vi "XY Graph Select Plots... Event.vi"(8 "Error In":errorcluster, 10 "Select (T)/Deselect":bool=TRUE, 11 "XYGraph Ref":T1) -> (0 "Error Out":errorcluster, 1 "Message":string, 2 "Plot Names":string[](array[string]), 3 "XYGraph Ref":T1, 5 "Graph Caption":string)   [LabVIEW 2021, in "XY Graph Add-Ons.lvlib"]
uses:
  XY Graph Add-Ons.lvlib
  XY Graph Refnum.ctl
  Time/Time.lvlib
  Strings/Strings.lvlib
panel:
  out "CPU (s)":dbl
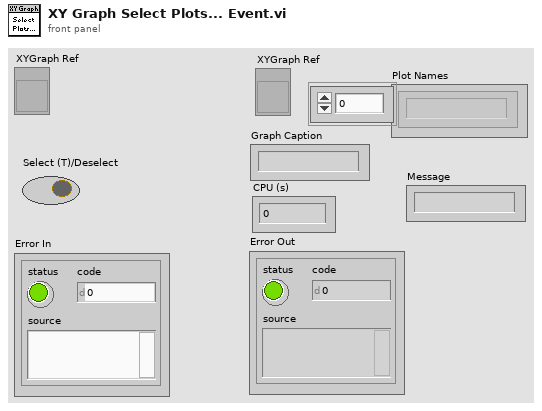
[diagram p1: front panel]
types:
  T1 = typedef "XY Graph Add-Ons.lvlib/XY Graph Refnum.ctl" = refnum<vi>
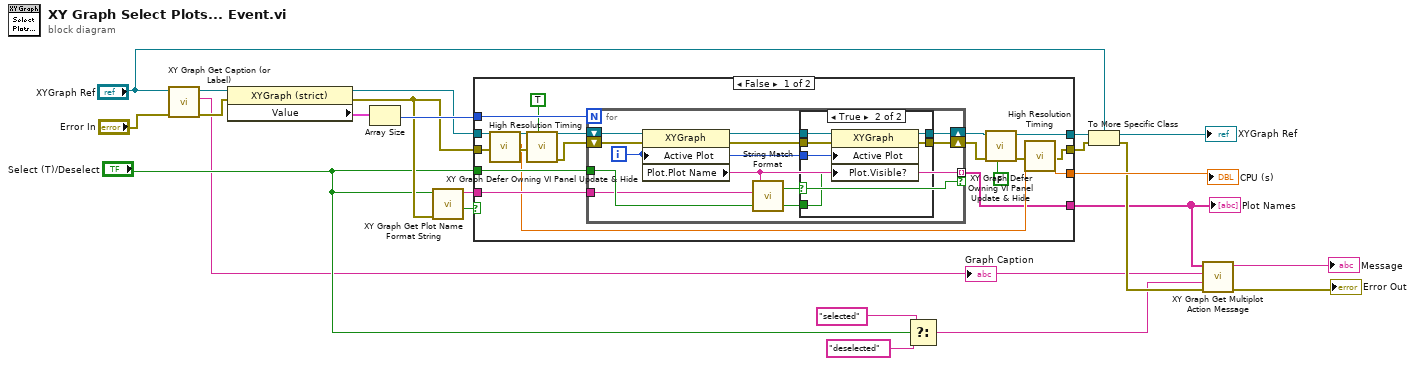
[diagram p0: block diagram]
diagram:
  n1 = call "XY Graph Get Caption (or Label).vi"("error in (no error)"="Error In", "XYGraph in"="XYGraph Ref") -> ("error out"=w2:errorcluster, "Caption (or Label) Text"=w1:string, "XYGraph out"=w4:T1)  [unwired: 7 in]
  "Graph Caption" <- w1
  n2 = property class="XYGraph (strict)"(reference=w4, error in=w2) -> (reference out=w21:T1, error out=w15:errorcluster, "Value"=w23:cluster{"X Array":dbl[], "Y Array":dbl[]}[])
  n3 = Array Size(array=w23) -> (size(s)=w22:i32)
  n4 = call "XY Graph Get Plot Name Format String.vi"("error in (no error)"=w15, "Select(T)/Deselect(F)"="Select (T)/Deselect") -> ("Cancelled?"=w16:bool, "String Format"=w17:string)  [unwired: 7 in, 1 out]
  n5 = case shown="False" w16 {
    tunnel: w22 -> [w41 _]
    tunnel: w21 -> [w40 w62]
    tunnel: [w35 w62] -> w20
    tunnel: [w26 w61] -> w18
    tunnel: w17 -> [w33 _]
    tunnel: "Select (T)/Deselect" -> [w32 _]
    tunnel: w15 -> [w29 w61]
    tunnel: [w27 _] -> w14
    tunnel: [w24 _] -> w11
    frame False {
      n6 = call "High Resolution Timing.vi"("Error In"=w29) -> ("elapsed (relative) seconds"=w25:dbl, "Error Out"=w28:errorcluster)  [unwired: 16 in, 1 out]
      n7 = call "XY Graph Defer Owning VI Panel Update & Hide.vi"("Defer Owning Panel Update"=TRUE ("Hide (F)/Show (T) Graph"), "error in (no error)"=w28, "XY Graph Refnum in"=w40) -> ("error out"=w38:errorcluster, "XY Graph Refnum out"=w39:refnum<vi>)  [unwired: 7 in]
      n8 = for {
        N: w41 -> [_]
        shift-right: [w52] -> w37
        shift-left: w39 -> [w49]
        shift-right: [w51] -> w36
        shift-left: w38 -> [w48]
        tunnel: w32 -> [w45]
        tunnel: w33 -> [w44]
        tunnel: [w43] -> w24 mode=indexing if=w42
        i -> [w50]
        n9 = property class="XYGraph"(reference=w49, error in=w48, "Active Plot"=w50) -> (reference out=w47:refnum<vi>, error out=w46:errorcluster, "Plot.Plot Name"=w43:string)
        n10 = call "String Match Format.vi"("String Format"=w44, "String"=w43) -> ("Match format?"=w42:bool)  [unwired: 3 in]
        n11 = case shown="True" w42 {
          tunnel: [w54 w60] -> w52
          tunnel: [w53 w59] -> w51
          tunnel: w50 -> [_ w58]
          tunnel: w47 -> [w54 w57]
          tunnel: w46 -> [w53 w56]
          tunnel: w45 -> [_ w55]
          frame False {
          }
          frame True {
            n12 = property class="XYGraph"(reference=w57, error in=w56, "Active Plot"=w58, "Plot.Visible?"=w55) -> (reference out=w60:refnum<vi>, error out=w59:errorcluster)
          }
        }
      }
      n13 = call "XY Graph Defer Owning VI Panel Update & Hide.vi"("Defer Owning Panel Update"=FALSE ("Hide (F)/Show (T) Graph"), "error in (no error)"=w36, "XY Graph Refnum in"=w37) -> ("error out"=w34:errorcluster, "XY Graph Refnum out"=w35:refnum<vi>)  [unwired: 7 in]
      n14 = call "High Resolution Timing.vi"("relative seconds (NaN)"=w25, "Error In"=w34) -> ("elapsed (relative) seconds"=w27:dbl, "Error Out"=w26:errorcluster)  [unwired: 15 in, 1 out]
    }
    frame True {
    }
  }
  "CPU (s)" <- w14
  "Plot Names" <- w11
  n15 = Select(t="selected" ("Graph Action"), s="Select (T)/Deselect", f="deselected" ("input 1")) -> (s? t:f=w6:string)
  n16 = To More Specific Class(target class="XYGraph Ref", reference=w20, error in=w18) -> (specific class reference=→"XYGraph Ref":T1, error out=w13:errorcluster)
  n17 = call "XY Graph Get Multiplot Action Message.vi"("error in (no error)"=w13, "Graph Action"=w6, "Graph Caption"=w1, "Plot Names"=w11) -> ("Error Out"=→"Error Out":errorcluster, "Multiplot Message"=→"Message":string)  [unwired: 6 in]
